vi "Updater Convert All TDMS Files 4.3 to 5.0.vi"(8 "error in (no error)":errorcluster, 10 "Map IndexName to FieldId":T1(array[cluster]), 11 "Folder Path":path) -> (0 "error out":errorcluster)   [LabVIEW 2011]
panel:
  in  "Continue":bool
  out "Estimated Time to Completion (min)":dbl format="%.2g"
  out "Avg Time Per File (sec)":dbl format="%.2g"
  out "Conversion Progress":u8(slide) max=21 scale=0.0..100.0
  out "Errors":string
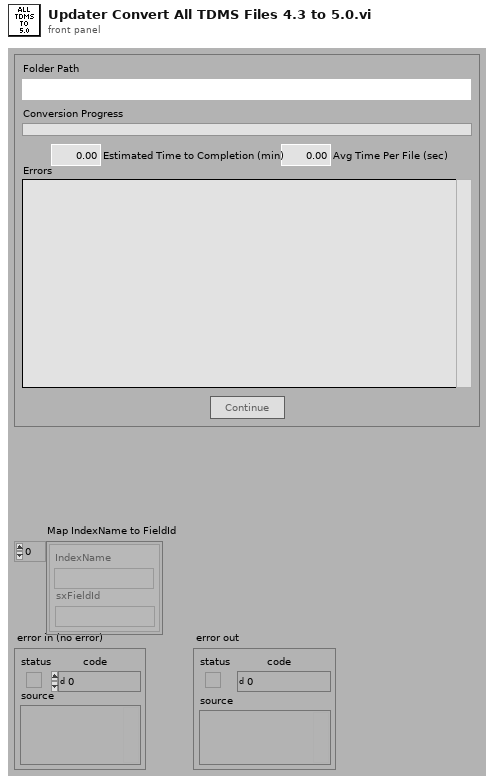
[diagram p1: front panel]
types:
  T1 = cluster{"IndexName":string, "sxFieldId":string}[]
  T2 = cluster{"left":i16, "top":i16, "right":i16, "bottom":i16}
  T3 = enum8{"Enabled", "Disabled", "Disabled and Grayed Out"}
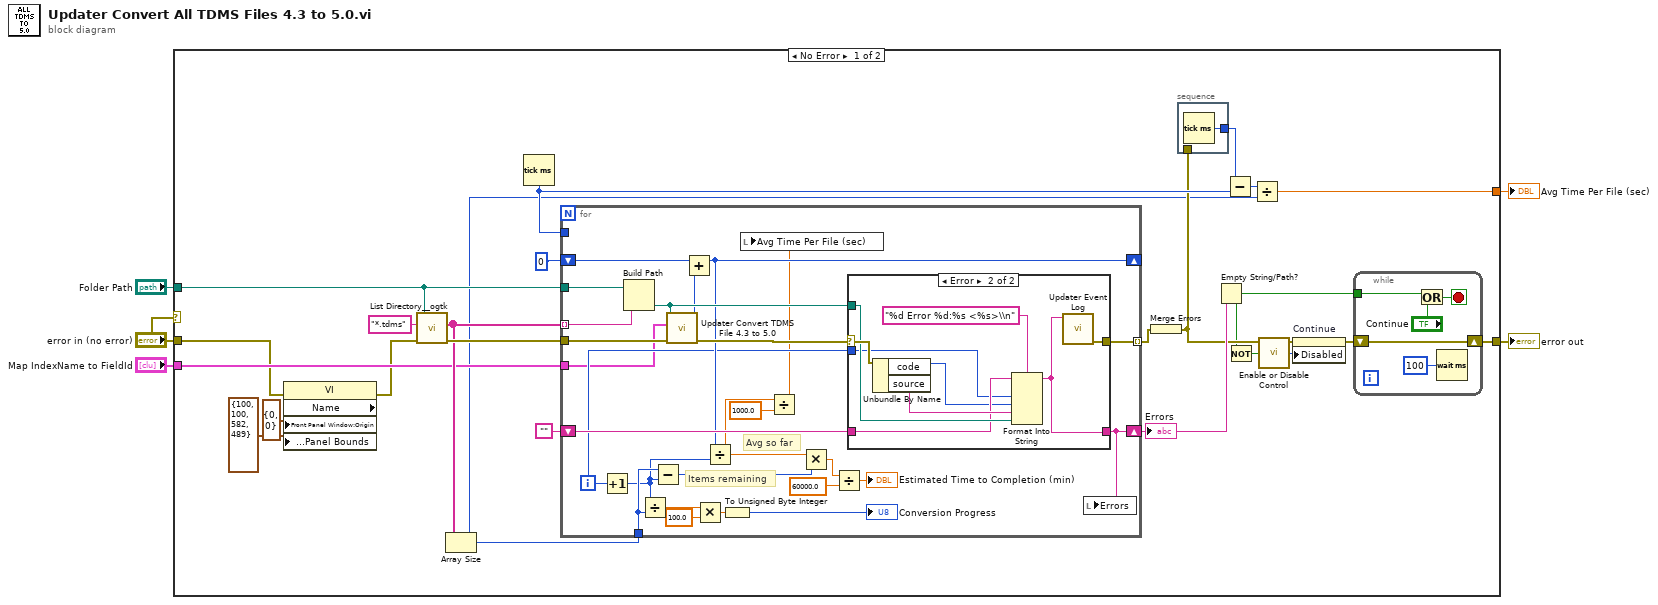
[diagram p0: block diagram]
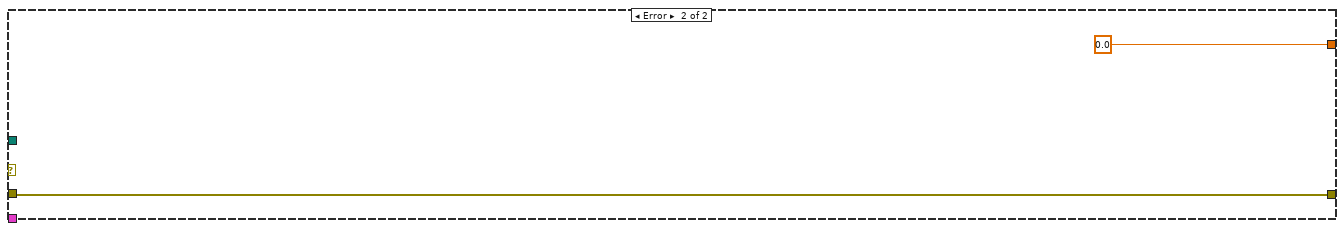
[diagram p3: hidden frame]
diagram:
  n1 = case shown="No Error" "error in (no error)" {
    tunnel: "error in (no error)" -> [w16 w74]
    tunnel: [w14 w74] -> w1
    tunnel: [w6 0.0] -> w5
    tunnel: "Folder Path" -> [w23 _]
    tunnel: "Map IndexName to FieldId" -> [w20 _]
    frame No Error {
      n2 = property class="VI" props=["Name", "Front Panel Window:Origin", "Front Panel Window:Panel Bounds"](error in=w16, "Front Panel Window:Origin"=cluster{"Horizontal":i16, "Vertical":i16} {"Horizontal"=0, "Vertical"=0}, "Front Panel Window:Panel Bounds"=T2 {"left"=100, "top"=100, "right"=582, "bottom"=489}) -> (error out=w15:errorcluster)  [unwired: 1 in, 2 out]
      n3 = call "List Directory__ogtk.vi"("error in (no error)"=w15, "pattern"="*.tdms", "directory path"=w23) -> ("error out"=w28:errorcluster, "file names"=w26:string[])  [unwired: 3 out]
      n4 = Array Size(array=w26) -> (size(s)=w7:i32)
      n5 = Tick Count (ms)() -> (millisecond timer value=w19:u32)
      n6 = for {
        tunnel: w23 -> [w61]
        tunnel: w26 -> [w60] mode=indexing
        tunnel: w28 -> [w59]
        tunnel: [w53] -> w27 mode=indexing
        tunnel: w7 -> [w48]
        shift-right: [w40] -> w13
        shift-left: "" -> [w51]
        shift-right: [w43] -> _
        shift-left: u32 0 ("y") -> [w50]
        tunnel: w20 -> [w39]
        tunnel: w19 -> [_]
        i -> [w41]
        # "Avg so far"
        # "Items remaining"
        n7 = Increment(x=w41) -> (x+1=w42:i32)
        n8 = Build Path(base path=w61, name or relative path=w60) -> (appended path=w52:path)
        n9 = Divide(x=w42, y=w48) -> (x/y=w58:dbl)
        n10 = Subtract(x=w48, y=w42) -> (x-y=w47:i32)
        n11 = call "Updater Convert TDMS File 4.3 to 5.0.vi"("error in (no error)"=w59, "Map IndexName to FieldId"=w39, "TDMS Path"=w52) -> ("error out"=w54:errorcluster, "Conversion Time (ms)"=w49:u32)  [unwired: 7 out]
        n12 = Add(x=w50, y=w49) -> (x+y=w43:u32)
        n13 = Multiply(x=w58, y=100.0) -> (x*y=w56:dbl)
        n14 = Divide(x=w43, y=w42) -> (x/y=w37:dbl)
        n15 = To Unsigned Byte Integer(number=w56) -> (unsigned 8bit integer=→"Conversion Progress":u8)
        n16 = Divide(x=w37, y=1000.0) -> (x/y=w36:dbl)
        n17 = local write "Avg Time Per File (sec)"(w36) -> ()
        n18 = Multiply(x=w37, y=w47) -> (x*y=w46:dbl)
        n19 = Divide(x=w46, y=60000.0) -> (x/y=→"Estimated Time to Completion (min)":dbl)
        n20 = case shown="Error" w54 {
          selector: w54 -> [w63 w72]
          tunnel: [w63 w65] -> w53
          tunnel: w52 -> [_ w70]
          tunnel: w51 -> [w62 w69]
          tunnel: [w62 w64] -> w40
          tunnel: w41 -> [_ w66]
          frame No Error {
          }
          frame Error {
            n21 = Unbundle By Name(w72) -> ("code"=w67:i32, "source"=w71:string)
            n22 = Format Into String(format string="%d Error %d:%s <%s>\\n" ("pattern"), initial string=w69, w66, w67, w71, w70) -> (resulting string=w64:string)  [unwired: 1 in, 1 out]
            n23 = call "Updater Event Log.vi"("Log Entry"=w64) -> ("error out"=w65:errorcluster)  [unwired: 1 in, 9 out]
          }
        }
        n24 = local write "Errors"(w40) -> ()
      }
      "Errors" <- w13
      n25 = Merge Errors(w27) -> (w12:errorcluster)
      n26 = stacked-sequence {
        tunnel: w12 -> [_]
        tunnel: [w35] -> w25
        frame #0 {
          n27 = Tick Count (ms)() -> (millisecond timer value=w35:u32)
        }
      }
      n28 = Empty String/Path?(string/path=w13) -> (empty?=w9:bool)
      n29 = Subtract(x=w25, y=w19) -> (x-y=w24:u32)
      n30 = Not(x=w9) -> (.not. x?=w8:bool)
      n31 = Divide(x=w24, y=w7) -> (x/y=w6:dbl)
      n32 = call "Enable or Disable Control.vi"("Enable? (T)"=w8) -> ("Enable\\Disable"=w10:T3)
      n33 = property on="Continue" class="Bool"(error in=w12, "Disabled"=w10) -> (error out=w11:errorcluster)  [unwired: 1 in, 1 out]
      n34 = while {
        shift-right: [w34] -> w14
        shift-left: w11 -> [w34]
        tunnel: w9 -> [w32]
        stop <- w30 stop-if-true
        n35 = Or(x=w32, y="Continue") -> (x .or. y?=w30:bool)
        n36 = Wait (ms)(milliseconds to wait=u32 100) -> ()  [unwired: 1 out]
      }
    }
    frame Error {
    }
  }
  "error out" <- w1
  "Avg Time Per File (sec)" <- w5
